vi "users file name.vi"() -> (8 "file name":string)   [LabVIEW 2012]
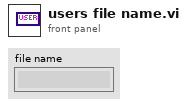
[diagram p1: front panel]
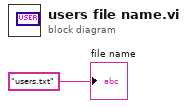
[diagram p0: block diagram]
diagram:
  "file name" <- "users.txt" ("file name")
